vi "Gather Test Data.vi"(0 "Agilent Scan List":string="101,102,103,104,105,106,107,108,109,110,111,112,113,114,115,116", 1 "Semiphore":T1, 2 "Equipment":T4={"COM Port"="COM1", "MW100"="MW100", "AG34970"="A-34972A", "WT500"="WT500"}, 5 "Tank Display Ref":refnum<vi>, 11 "error in (no error)":errorcluster) -> (6 "Output Data":string[][](array[string]), 15 "error out":errorcluster={"status"=TRUE, "code"=-1073807346, "source"="VISA Read in Gather Test Data.vi"})   [LabVIEW 2009]
uses:
  <instrlib>/Agilent 34970/Agilent 34970.lvlib
  ChannelSettings.ctl
  EquipReferences.ctl
  HEWH Tank Indicator.ctl
panel:
  out "Tambient":dbl
  in  "COM Port Timeout Value":u32=10000
  out "34970 Data":string[](array[string])=["32.000000E+0"]
  out "Power Data":string[](array[string])=["0.000000E+0", "0.000000E+0", "0.000000E+0", "0.000000E+0"]
  out "PowerData":T2
  out "Local Tank Display":T3 {"TIN" format="%.2g"; "TOUT" format="%.2g"; "Mean" format="%.2f"; "Std Dev" format="%.2f"; "TC6" format="%.2g"; "TC5" format="%.2g"; "TC4" format="%.2g"; "TC3" format="%.2g"; "TC2" format="%.2g"; "TC1" format="%.2g"}
  out "MW100 Data":string[](array[string])=["0.000000E+0", "0.000000E+0"]
  out "Serial Data":string
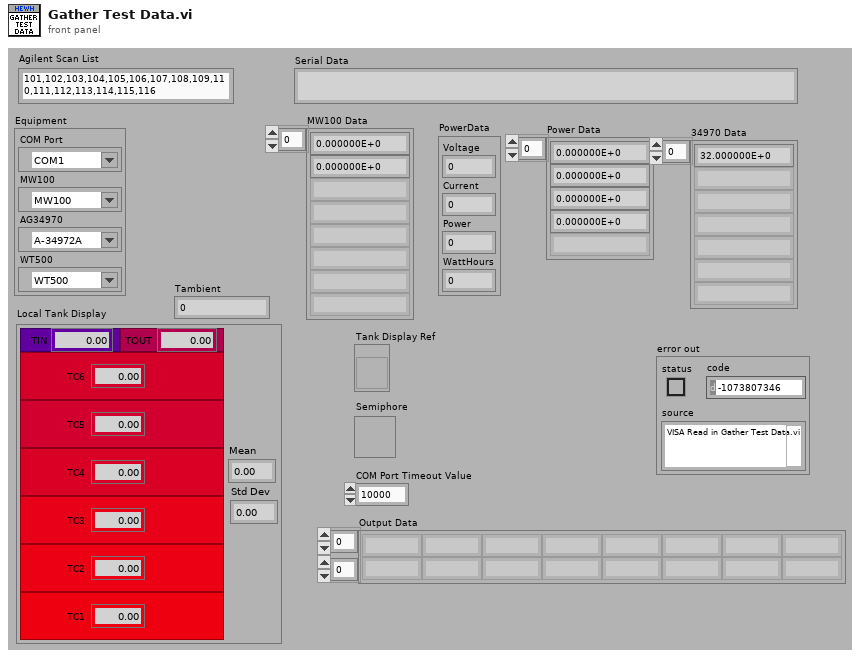
[diagram p1: front panel]
types:
  T1 = typedef "Semaphore RefNum" = refnum<k1>
  T2 = cluster{"Voltage":dbl, "Current":dbl, "Power":dbl, "WattHours":dbl}
  T3 = typedef "HEWH Tank Indicator.ctl" = cluster{"TC1-D":bool, "TC2-D":bool, "TC3-D":bool, "TC4-D":bool, "TC5-D":bool, "TC6-D":bool, "RTD_IN":bool, "RTDOUT":bool, "TC1":dbl, "TC2":dbl, "TC3":dbl, "TC4":dbl, "TC5":dbl, "TC6":dbl, "TIN":dbl, "TOUT":dbl, "Std Dev":dbl, "Mean":dbl}
  T4 = typedef "EquipReferences.ctl" = cluster{"COM Port":refnum<visa-resource-name>, "MW100":refnum<visa-resource-name>, "AG34970":refnum<visa-resource-name>, "WT500":refnum<visa-resource-name>}
  T5 = typedef "ChannelSettings.ctl" = u16
  T6 = typedef "PowerData.ctl" = cluster{"Voltage":dbl, "Current":dbl, "Power":dbl, "WattHours":dbl}
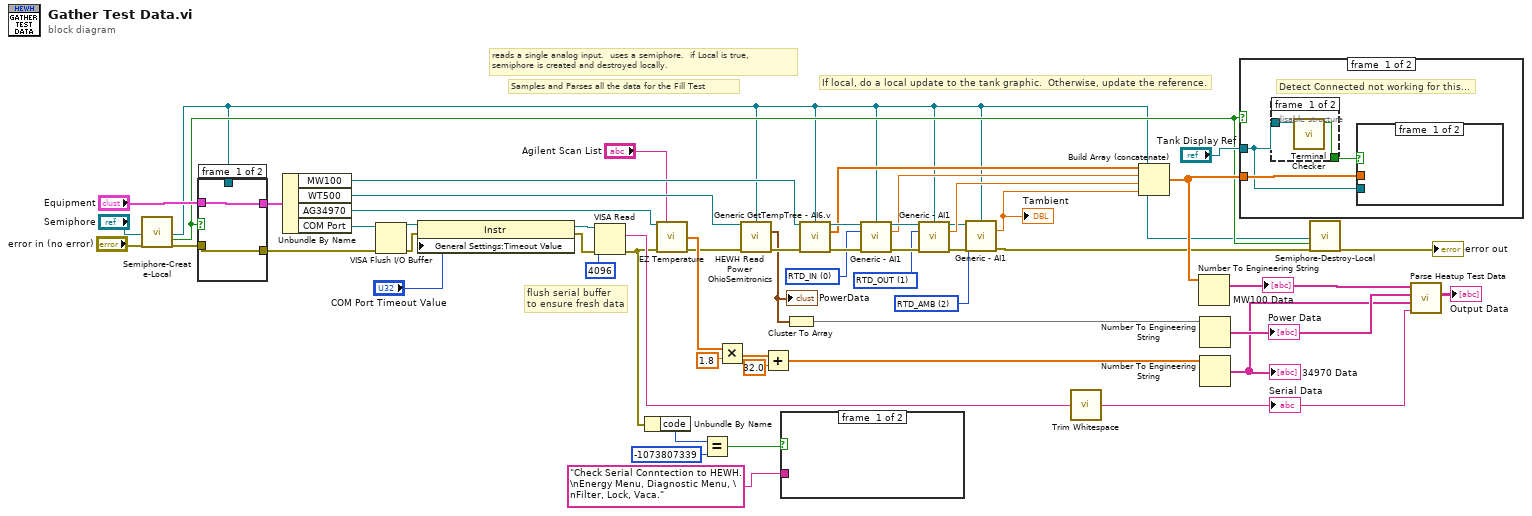
[diagram p0: block diagram]
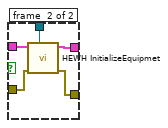
[diagram p2: hidden frame]
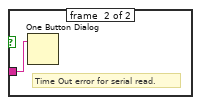
[diagram p3: hidden frame]
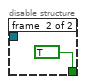
[diagram p4: hidden frame]
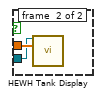
[diagram p5: hidden frame]
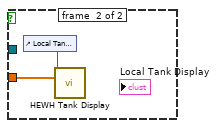
[diagram p6: hidden frame]
diagram:
  w4 = T5 2 items=["RTD_IN", "RTD_OUT", "RTD_AMB", "Tc_1", "Tc_2", "Tc_3", "Tc_4", "Tc_5", "Tc_6", "Tc_down", "Pres_HI1", "Pres_HI2", "Pres_LOW", "VLV_IN", "VLV_DUMP", "VLV_OUT", "PWR_MAIN", "FLOWMETER", "4-20_OUT", "HEATER_TOP", "HEATER_BOT", "Pres_H2OIn", "DRM_LOW", "DRM_HIGH", "INTF_TEMPFLO", "INTF_READY", "INTF_START", "INTF_STOP"] ("Channel_Enum")
  w26 = T5 0 items=["RTD_IN", "RTD_OUT", "RTD_AMB", "Tc_1", "Tc_2", "Tc_3", "Tc_4", "Tc_5", "Tc_6", "Tc_down", "Pres_HI1", "Pres_HI2", "Pres_LOW", "VLV_IN", "VLV_DUMP", "VLV_OUT", "PWR_MAIN", "FLOWMETER", "4-20_OUT", "HEATER_TOP", "HEATER_BOT", "COMPRESSOR", "DRM_LOW", "DRM_HIGH", "INTF_TEMPFLO", "INTF_READY", "INTF_START", "INTF_STOP"] ("Channel_Enum")
  w27 = T5 1 items=["RTD_IN", "RTD_OUT", "RTD_AMB", "Tc_1", "Tc_2", "Tc_3", "Tc_4", "Tc_5", "Tc_6", "Tc_down", "Pres_HI1", "Pres_HI2", "Pres_LOW", "VLV_IN", "VLV_DUMP", "VLV_OUT", "PWR_MAIN", "FLOWMETER", "4-20_OUT", "HEATER_TOP", "HEATER_BOT", "COMPRESSOR", "DRM_LOW", "DRM_HIGH", "INTF_TEMPFLO", "INTF_READY", "INTF_START", "INTF_STOP"] ("Channel_Enum")
  # "reads a single analog input.  uses a semiphore.  if Local is true, \nsemiphore is created and destroyed locally."
  # "If local, do a local update to the tank graphic.  Otherwise, update the reference."
  # "flush serial buffer\nto ensure fresh data"
  # "Samples and Parses all the data for the Fill Test"
  n1 = call "Semiphore-Create-Local.vi"("Semiphore"="Semiphore", "error in (no error)"="error in (no error)") -> ("semaphore"=w1:T1, "Local?"=w8:bool, "error out"=w11:errorcluster)  [unwired: 15 in]
  n2 = case shown="True" w8 {
    tunnel: [w58 w62] -> w13
    tunnel: "Equipment" -> [w58 w63]
    tunnel: w11 -> [w57 w61]
    tunnel: [w57 w60] -> w10
    tunnel: w1 -> [_ w59]
    frame #0 {
    }
    frame #1 {
      n3 = call "HEWH InitializeEquipmet.vi"("Semiphore"=w59, "Error In"=w61, "Equipment"=w63) -> ("Error Out"=w60:errorcluster, "Equipment Out"=w62:T4)  [unwired: 7 in]
    }
  }
  n4 = Unbundle By Name(w13) -> ("MW100"=w53:refnum<visa-resource-name>, "WT500"=w56:refnum<visa-resource-name>, "AG34970"=w39:refnum<visa-resource-name>, "COM Port"=w30:refnum<visa-resource-name>)
  n5 = VISA Flush I/O Buffer(VISA resource name=w30, error in (no error)=w10) -> (VISA resource name out=w20:refnum<visa-resource-name>, error out=w17:errorcluster)  [unwired: 1 in]
  n6 = property class="Instr"(reference=w20, error in=w17, "General Settings:Timeout Value"="COM Port Timeout Value") -> (reference out=w19:refnum<visa-resource-name>, error out=w18:errorcluster)
  n7 = VISA Read(VISA resource name=w19, byte count=u32 4096, error in (no error)=w18) -> (read buffer=w31:string, error out=w24:errorcluster)  [unwired: 2 out]
  n8 = Unbundle By Name(w24) -> ("code"=w23:i32)
  n9 = call <instrlib>:"EZ Temperature.vi"("VISA Resource Name"=w39, "Scan List (empty)"="Agilent Scan List", "error in (no error)"=w24) -> ("Output Array"=w41:dbl[], "error out"=w40:errorcluster)  [unwired: 10 in, 1 out]
  n10 = Equal?(x=w23, y=-1073807339 ("code")) -> (x = y?=w25:bool)
  n11 = Multiply(x=w41, y=1.8) -> (x*y=w43:dbl[])
  n12 = call "HEWH Read Power OhioSemitronics.vi"("VISA resource name"=w56, "Semiphore"=w1, "error in (no error)"=w40) -> ("PowerData"=w2:T6, "error out"=w29:errorcluster)  [unwired: 9 in, 2 out]
  "PowerData" <- w2
  n13 = Add(x=w43, y=32.0) -> (x+y=w37:dbl[])
  n14 = case shown="True" w25 {
    tunnel: "Check Serial Conntection to HEWH.\nEnergy Menu, Diagnostic Menu, \nFilter, Lock, Vaca." ("error source (\" \")") -> [_ w64]
    frame #0 {
    }
    frame #1 {
      # "Time Out error for serial read."
      n15 = One Button Dialog(message=w64) -> ()  [unwired: 1 in, 1 out]
    }
  }
  n16 = Cluster To Array(cluster=w2) -> (array=w45:dbl[])
  n17 = call "Generic GetTempTree - AI6.v.vi"("MW100"=w53, "Semiphore"=w1, "Error In"=w29) -> ("dup VISA session"=w49:refnum<visa-resource-name>, "Tc Tree"=w48:dbl[], "error out"=w52:errorcluster)  [unwired: 10 in]
  n18 = call "Generic - AI1.vi"("MW100"=w49, "Semiphore"=w1, "Channel_Enum"=w26, "Error In"=w52) -> ("dup VISA session"=w51:refnum<visa-resource-name>, "Value"=w47:dbl, "Error Out"=w50:errorcluster)  [unwired: 9 in]
  n19 = call "Generic - AI1.vi"("MW100"=w51, "Semiphore"=w1, "Channel_Enum"=w27, "Error In"=w50) -> ("dup VISA session"=w7:refnum<visa-resource-name>, "Value"=w46:dbl, "Error Out"=w6:errorcluster)  [unwired: 9 in]
  n20 = call "Generic - AI1.vi"("MW100"=w7, "Semiphore"=w1, "Channel_Enum"=w4, "Error In"=w6) -> ("Value"=w3:dbl, "Error Out"=w5:errorcluster)  [unwired: 9 in, 1 out]
  "Tambient" <- w3
  n21 = call <vilib>:"Trim Whitespace.vi"("string"=w31) -> ("trimmed string"=w32:string)  [unwired: 1 in]
  "Serial Data" <- w32
  n22 = Build Array (concatenate)(w48, w47, w46, w3) -> (w33:dbl[])
  n23 = Number To Engineering String(4:w33) -> (0:w55:string[])  [unwired: 3 in]
  "MW100 Data" <- w55
  n24 = Number To Engineering String(4:w45) -> (0:w36:string[])  [unwired: 3 in]
  "Power Data" <- w36
  n25 = Number To Engineering String(4:w37) -> (0:w35:string[])  [unwired: 3 in]
  "34970 Data" <- w35
  n26 = case shown="False" w8 {
    tunnel: w33 -> [w67 w74]
    tunnel: "Tank Display Ref" -> [w65 _]
    frame #0 {
      # "Detect Connected not working for this..."
      n27 = disable-structure shown="Enabled" {
        disable-tunnel: [w69 TRUE ("is connected?")] -> w66
        disable-tunnel: w65 -> [w68 _]
        frame #0 {
          n28 = call "Terminal Checker.vi"("control reference"=w68) -> ("is connected?"=w69:bool)  [unwired: 9 in, 1 out]
        }
        frame #1 {
        }
      }
      n29 = case shown="True" w66 {
        tunnel: w67 -> [_ w72]
        tunnel: w65 -> [_ w71]
        frame #0 {
        }
        frame #1 {
          n30 = call "HEWH Tank Display.vi"("Local Tank Display"=w71, "T1-T6.Tin,Tout"=w72) -> ()  [unwired: 13 in, 1 out]
        }
      }
    }
    frame #1 {
      n31 = control-ref of="Local Tank Display"() -> (w73:refnum<vi>)
      n32 = call "HEWH Tank Display.vi"("Local Tank Display"=w73, "T1-T6.Tin,Tout"=w74) -> ()  [unwired: 13 in, 1 out]
    }
  }
  n33 = call "Semiphore-Destroy-Local.vi"("Semiphore"=w1, "Local?"=w8, "error in (no error)"=w5) -> ("error out"=→"error out":errorcluster)  [unwired: 16 in]
  n34 = call "Parse Heatup Test Data.vi"("Serial Data"=w32, "34970 Data"=w35, "WT500 Data"=w36, "MW100 Data"=w55) -> ("Output Data"=→"Output Data":string[][])  [unwired: 7 in]
